vi "Plan.vi"(0 "Response Case":T2, 1 "Caller in":refnum<class "Worker.lvclass">, 2 "Auxiliary":variant, 5 "Data":variant, 7 "Timeout (1000ms)":u32=1000, 9 "Continius? (F)":bool, 11 "error in (no error)":errorcluster, 12 "Time Precission (100ms)":u32=100, 13 "Priority (Normal)":T1=enum."Normal", 14 "Debugger MSG? (F)":bool) -> (3 "dup Caller out":refnum<class "Worker.lvclass">, 4 "Work Planer out":refnum<class "Work Planer.lvclass">, 15 "error out":errorcluster)   [LabVIEW 2018, in "Work Planer.lvclass"]
uses:
  Work Planer.lvclass
  <vilib>/addons/_Workers/Library/Classes/Worker/Worker.lvclass
  <vilib>/addons/_Workers/Library/Case Label.ctl
  <vilib>/addons/_Workers/Library/Classes/Message/Priority (ALL).ctl
  Initialization Data.ctl
  Response Cases.ctl
  <vilib>/addons/_Workers/Library/Workers.lvlib
  <vilib>/addons/_Workers/Library/Classes/Message/Message.lvclass
panel:
  out "concatenated string":string
  in  "Worker Alias":string="Work Planer "
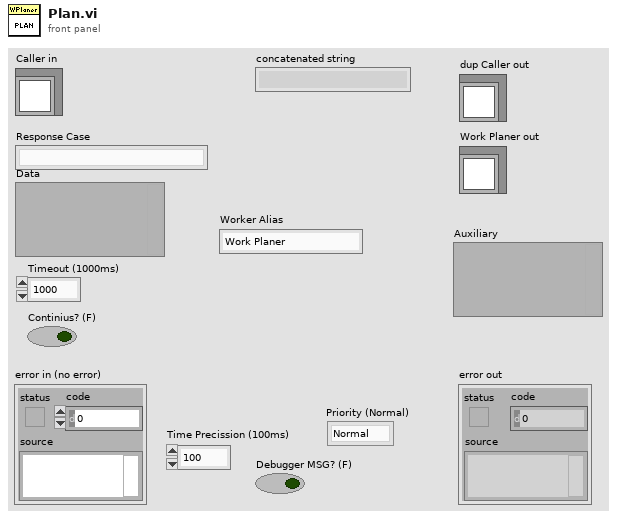
[diagram p1: front panel]
types:
  T1 = typedef "Workers.lvlib/Message.lvclass/Priority (ALL).ctl" = enum16{"Low", "Normal", "High", "Critical"}
  T2 = typedef "Workers.lvlib/Case Label.ctl" = string
  T3 = typedef "Work Planer.lvclass/Initialization Data.ctl" = cluster{"Response Cases":T4, "Time Precission (100ms)":u32, "Continius? (F)":bool, "Data":variant, "Auxiliary":variant, "Priority (Normal)":T1, "Timeout (1000ms)":u32, "Debugger MSG? (T)":bool}
  T4 = typedef "Work Planer.lvclass/Response Cases.ctl" = cluster{"Timeout":T2}
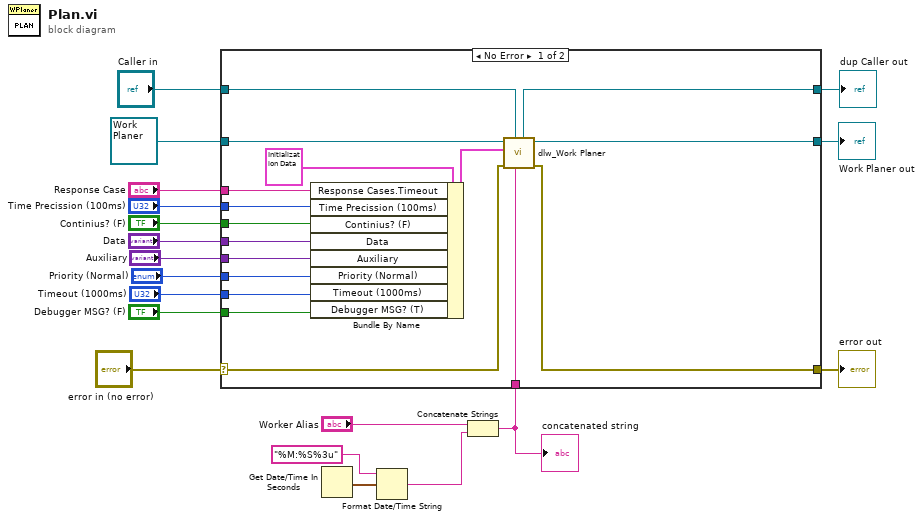
[diagram p0: block diagram]
diagram:
  n1 = Get Date/Time In Seconds() -> (seconds since 1Jan1904=w4:timestamp)
  n2 = Format Date/Time String(time format string (%c)="%M:%S%3u", seconds (now)=w4) -> (date/time string=w3:string)  [unwired: 1 in]
  n3 = Concatenate Strings("Worker Alias", w3) -> (w5:string)
  "concatenated string" <- w5
  n4 = case shown="No Error" "error in (no error)" {
    selector: "error in (no error)" -> [w30 w39]
    tunnel: [w29 w39] -> w18
    tunnel: [w35 w38] -> w16
    tunnel: refnum<class "Work Planer.lvclass"> refnum ("Work Planer in") -> [w36 w38]
    tunnel: "Caller in" -> [w34 w37]
    tunnel: [w33 w37] -> w14
    tunnel: "Continius? (F)" -> [w28 _]
    tunnel: "Time Precission (100ms)" -> [w27 _]
    tunnel: "Auxiliary" -> [w26 _]
    tunnel: "Debugger MSG? (F)" -> [w25 _]
    tunnel: "Timeout (1000ms)" -> [w24 _]
    tunnel: "Priority (Normal)" -> [w23 _]
    tunnel: "Data" -> [w22 _]
    tunnel: w5 -> [w21 _]
    tunnel: "Response Case" -> [w20 _]
    frame No Error {
      n5 = Bundle By Name(cluster=T3 {"Response Cases"={"Timeout"=""}, "Time Precission (100ms)"=100, "Continius? (F)"=FALSE, "Data"=variant, "Auxiliary"=variant, "Priority (Normal)"=enum."Normal", "Timeout (1000ms)"=1000, "Debugger MSG? (T)"=TRUE} ("Initialization Data"), "Response Cases.Timeout"=w20, "Time Precission (100ms)"=w27, "Continius? (F)"=w28, "Data"=w22, "Auxiliary"=w26, "Priority (Normal)"=w23, "Timeout (1000ms)"=w24, "Debugger MSG? (T)"=w25) -> (w31:T3)
      n6 = call "dlw_Work Planer.vi"("Worker Alias"=w21, "Caller in"=w34, "error in"=w30, "Initialization Data"=w31, "Work Planer in"=w36) -> ("error out"=w29:errorcluster, "Work Planer out"=w35:refnum<class "Work Planer.lvclass">, "dup Caller out"=w33:refnum<class "Worker.lvclass">)  [unwired: 4 in]
    }
    frame Error {
    }
  }
  "error out" <- w18
  "Work Planer out" <- w16
  "dup Caller out" <- w14
